vi "to_json.vi"(8 "error in":errorcluster, 11 "timestampManifest in":refnum<class "timestampManifest.lvclass">) -> (0 "error out":errorcluster, 2 "json":string, 3 "timestampManifest out":refnum<class "timestampManifest.lvclass">, 4 "Not Default":bool)   [LabVIEW 2020, in "nominal types.lvlib" / "timestampManifest.lvlib" / "timestampManifest.lvclass"]
uses:
  timestampManifest.lvclass
  timestampManifest.lvclass/timestampManifest.ctl
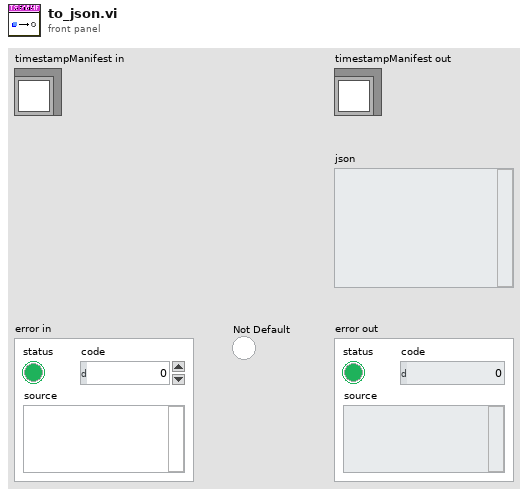
[diagram p1: front panel]
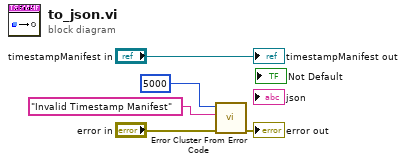
[diagram p0: block diagram]
diagram:
  n1 = call <vilib>:"Error Cluster From Error Code.vi"("error in (no error)"="error in", "error message (\"\")"="Invalid Timestamp Manifest" ("error message (\"\")"), "error code (0)"=5000) -> ("error out"=→"error out":errorcluster)  [unwired: 6 in]
  "timestampManifest out" <- "timestampManifest in"
